vi "Create Rooms Size Details Map.vi"(11 "error in (no error)":errorcluster) -> (4 "Rooms Size Details Map":map{string, T1}(c390), 15 "error out":errorcluster)   [LabVIEW 2023, in "File Data Manager.lvlib" / "File Data Manager.lvclass"]
uses:
  File Data Manager.lvclass
  Central Data Manager/Central Data Manager/Room Size Details.ctl
  <vilib>/Utility/file.llb/Read Delimited Spreadsheet (string).vi
  File Data Manager.lvclass/File Data Manager.ctl
  Utilities/Utilities.lvlib
  Central Data Manager/Central Data Manager/Central Data Manager.lvclass
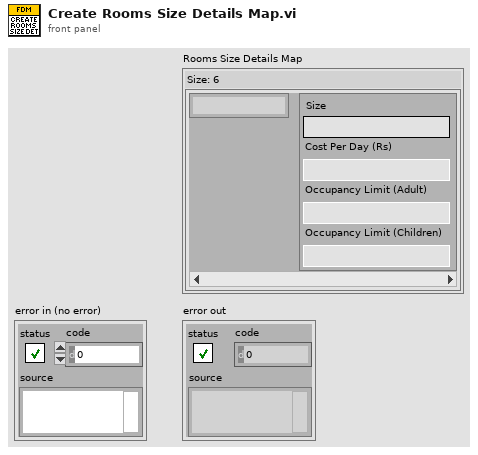
[diagram p1: front panel]
types:
  T1 = typedef "Central Data Manager.lvlib/Central Data Manager.lvclass/Room Size Details.ctl" = cluster{"Size":string, "Cost Per Day (Rs)":u32, "Occupancy Limit (Adult)":u32, "Occupancy Limit (Children)":u32}
  T2 = typedef "Hotel Management Tool Model.lvlib/Hotel Management Tool Model.lvclass/Database File Paths.ctl" = cluster{"Food Menu File Path":path, "Guests Histroy File Path":path, "Room Size File Path":path, "Rooms List File Path":path, "Rooms Service Allocation File Path":path, "Staff List File Path":path}
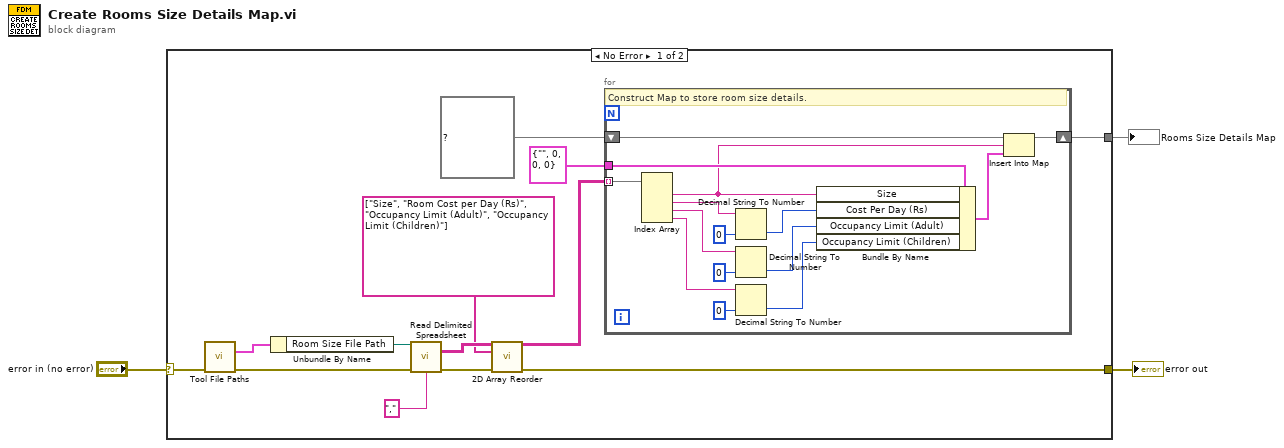
[diagram p0: block diagram]
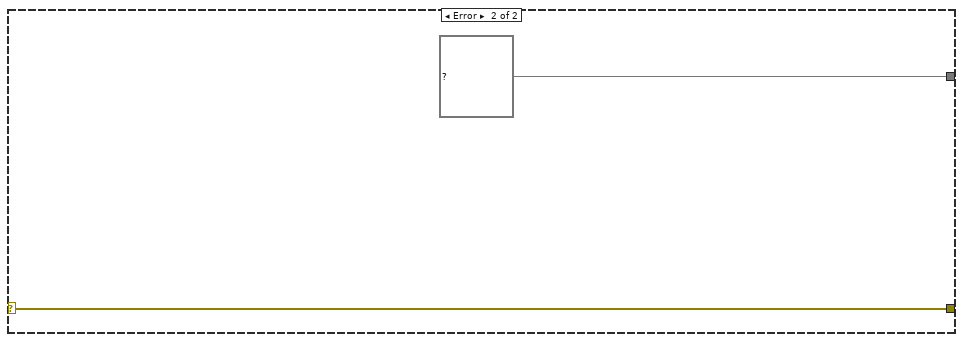
[diagram p2: hidden frame]
diagram:
  n1 = case shown="No Error" "error in (no error)" {
    selector: "error in (no error)" -> [w6 w33]
    tunnel: [w5 w33] -> w2
    tunnel: [w4 map{string, T1} {} ("Rooms Size Details")] -> w1
    frame No Error {
      n2 = call "Tool File Paths.vi"("error in (no error)"=w6) -> ("Database File Paths"=w16:T2, "error out"=w15:errorcluster)  [unwired: 12 in, 1 out]
      n3 = Unbundle By Name(w16) -> ("Room Size File Path"=w14:path)
      n4 = call-poly <vilib>:"Read Delimited Spreadsheet.vi"("file path (dialog if empty)"=w14, "error in (no error)"=w15, "delimiter (\\t)"="," ("delimiter (\\t)")) -> ("all rows"=w12:string[][], "error out"=w10:errorcluster)  [unwired: 7 in, 4 out]
      n5 = call "2D Array Reorder.vi"("2D Array Data witjh Header"=w12, "Header Order"=string[] ["Size", "Room Cost per Day (Rs)", "Occupancy Limit (Adult)", "Occupancy Limit (Children)"] ("first row"), "error in (no error)"=w10) -> ("Reordered Data without Header"=w9:string[][], "error out"=w5:errorcluster)  [unwired: 11 in]
      n6 = for {
        tunnel: w9 -> [w28] mode=indexing
        shift-right: [w30] -> w4
        shift-left: map{string, T1} {} ("Rooms Size Details") -> [w31]
        tunnel: T1 {"Size"="", "Cost Per Day (Rs)"=0, "Occupancy Limit (Adult)"=0, "Occupancy Limit (Children)"=0} ("value") -> [w29]
        # "Construct Map to store room size details."
        n7 = Index Array(array=w28) -> (element #1=w27:string, element #2=w23:string, element #3=w22:string, element #4=w21:string)  [unwired: 4 in]
        n8 = Decimal String To Number(string=w23, default (0L)=u32 0 ("Cost Per Day (Rs)")) -> (number=w18:u32)  [unwired: 1 in, 1 out]
        n9 = Decimal String To Number(string=w22, default (0L)=u32 0 ("Cost Per Day (Rs)")) -> (number=w19:u32)  [unwired: 1 in, 1 out]
        n10 = Decimal String To Number(string=w21, default (0L)=u32 0 ("Cost Per Day (Rs)")) -> (number=w20:u32)  [unwired: 1 in, 1 out]
        n11 = Bundle By Name(cluster=w29, "Size"=w27, "Cost Per Day (Rs)"=w18, "Occupancy Limit (Adult)"=w19, "Occupancy Limit (Children)"=w20) -> (w17:T1)
        n12 = Insert Into Map(map in=w31, key=w27, value=w17) -> (map out=w30:map{string, T1})  [unwired: 2 out]
      }
    }
    frame Error {
    }
  }
  "error out" <- w2
  "Rooms Size Details Map" <- w1
